vi "Value by Indices.vi"(8 "error in (no error)":errorcluster, 10 "Children Indices":i32[](array[numeric]), 11 "OpenHW in":refnum<class "OpenHW.lvclass">) -> (0 "error out":errorcluster, 2 "HW Node":T1, 3 "OpenHW out":refnum<class "OpenHW.lvclass">)   [LabVIEW 2022 SP3, in "open-hw-mon-lv.lvlib" / "OpenHW.lvclass"]
uses:
  OpenHW.lvclass
  HW Node.ctl
  OpenHW.lvclass/OpenHW.ctl
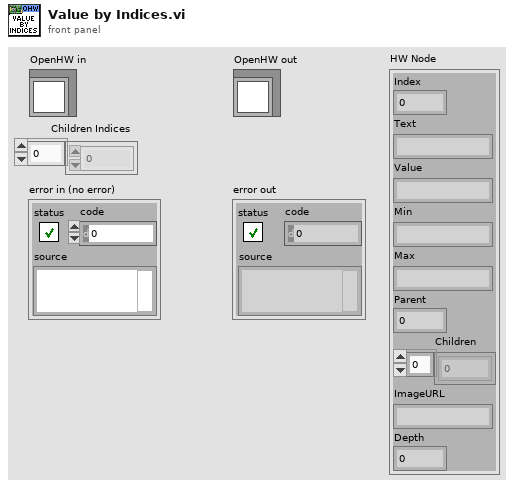
[diagram p1: front panel]
types:
  T1 = typedef "open-hw-mon-lv.lvlib/OpenHW.lvclass/HW Node.ctl" = cluster{"Index":i32, "Text":string, "Value":string, "Min":string, "Max":string, "Parent":i32, "Children":i32[], "ImageURL":string, "Depth":i32}
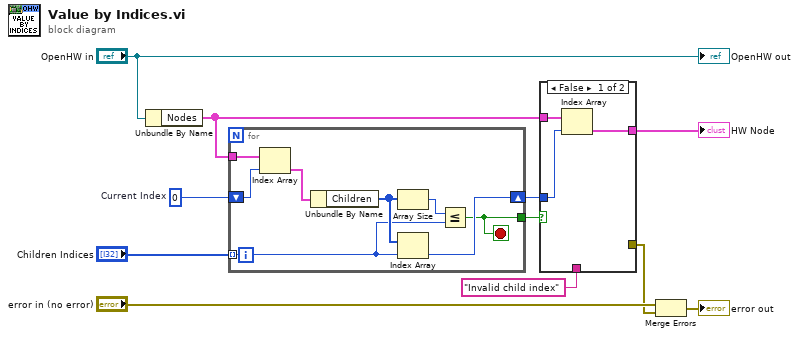
[diagram p0: block diagram]
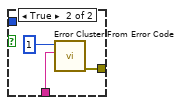
[diagram p2: hidden frame]
diagram:
  w9 = 0  # Current Index
  n1 = Unbundle By Name("OpenHW in") -> ("Nodes"=w6:T1[])
  n2 = for {
    tunnel: w6 -> [w19]
    tunnel: "Children Indices" -> [w14] mode=indexing
    shift-right: [w13] -> w7
    shift-left: w9 -> [w18]
    tunnel: [w12] -> w8
    stop <- w12 stop-if-true
    n3 = Index Array(array=w19, index=w18) -> (element=w17:T1)
    n4 = Unbundle By Name(w17) -> ("Children"=w15:i32[])
    n5 = Array Size(array=w15) -> (size(s)=w16:i32)
    n6 = Index Array(array=w15, index=w14) -> (element=w13:i32)
    n7 = Less Or Equal?(x=w16, y=w14) -> (x <= y?=w12:bool)
  }
  n8 = case shown="False" w8 {
    tunnel: w7 -> [w21 _]
    tunnel: w6 -> [w22 _]
    tunnel: [w20 _] -> w5
    tunnel: "Invalid child index" -> [_ w24]
    tunnel: [_ w23] -> w2
    frame False {
      n9 = Index Array(array=w22, index=w21) -> (element=w20:T1)
    }
    frame True {
      n10 = call <vilib>:"Error Cluster From Error Code.vi"("error message (\"\")"=w24, "error code (0)"=1) -> ("error out"=w23:errorcluster)  [unwired: 7 in]
    }
  }
  "HW Node" <- w5
  n11 = Merge Errors("error in (no error)", w2) -> (→"error out":errorcluster)
  "OpenHW out" <- "OpenHW in"
